vi "FG_ThreadInfo.vi"(7 "Command":enum16{"Set", "Get"}(ring)=enum."Get", 8 "error in (no error)":errorcluster, 11 "ThreadsStates":T1) -> (0 "error out":errorcluster, 3 "ThreadsStates Out":T1)   [LabVIEW 2012]
uses:
  #TD_ThreadsStates.ctl
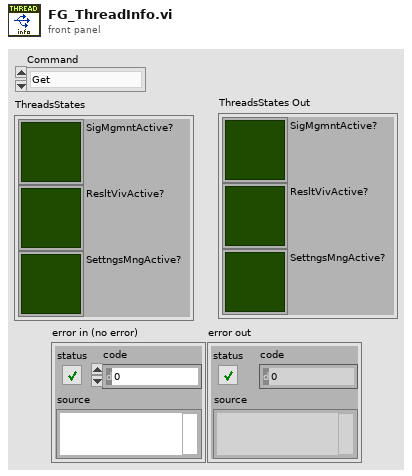
[diagram p1: front panel]
types:
  T1 = typedef "#TD_ThreadsStates.ctl" = cluster{"SigMgmntActive?":bool, "ResltVivActive?":bool, "SettngsMngActive?":bool}
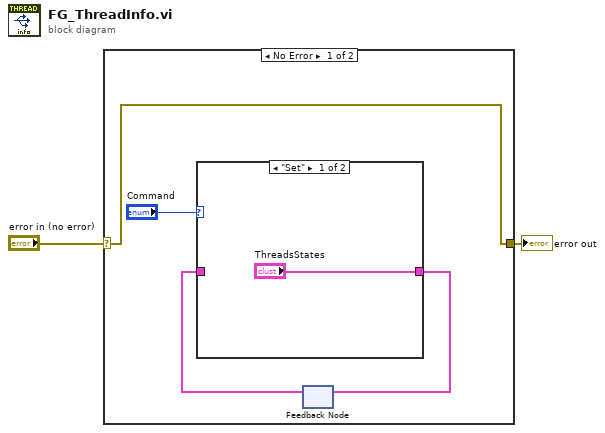
[diagram p0: block diagram]
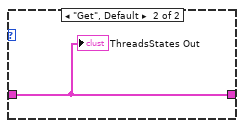
[diagram p2: hidden frame]
diagram:
  n1 = case shown="No Error" "error in (no error)" {
    selector: "error in (no error)" -> [w3 w9]
    tunnel: [w3 w9] -> w1
    frame No Error {
      n2 = feedback #1() -> (w4:T1)  [unwired: 1 in]
      n3 = case shown="\"Set\"" "Command" {
        tunnel: ["ThreadsStates" w8] -> w5
        tunnel: w4 -> [_ w8]
        frame "Set" {
        }
        frame "Get", Default {
          "ThreadsStates Out" <- w8
        }
      }
      n4 = feedback-in #1(w5) -> ()
    }
    frame Error {
    }
  }
  "error out" <- w1
